vi "LoggingProcess.vi"(0 "Buffers":T3, 5 "FPGA Ref":refnum<k20>, 7 "LoggingIRQ":i32, 11 "error in (no error)":errorcluster, 12 "AnalogLimits":T1) -> ()   [LabVIEW 2015]
uses:
  <vilib>/NI/PowerElectronicsControl/BufferLogging/Buffers.ctl
  <vilib>/NI/PowerElectronicsControl/ScaleAndLimit/Interface/Interface.ctl
  <instrlib>/_niInstr/Instruction Framework/v1/Host/Instruction Target/niInstr Instruction Target v1 Host.lvclass
  <instrlib>/_niInstr/Instruction Framework/v1/Host/Instruction Framework Context/niInstr Instruction Framework Context v1 Host.lvclass
  <vilib>/NI/PowerElectronicsControl/ScaleAndLimit/Interface/Configuration.ctl
  <vilib>/Utility/error.llb/Error Cluster From Error Code.vi
  <vilib>/RVI Host/nirviSupport.llb/nirviErrorClusterFromErrorCode.vi
  <vilib>/rvi/errors/niLvFpgaAdjustHostInterfaceError.vi
  <vilib>/rvi/interface/nirviMethod/nirviMethod.xnode
  <vilib>/rvi/interface/nirviReadWriteControl/nirviReadWriteControl.xnode
  <vilib>/NI/PowerElectronicsControl/BufferLogging/BufferLogging.lvlib
  <vilib>/rvi/interface/nirviMethod/StockFPGA_InlinedMethodWaitForSingleIRQ.vi
  <vilib>/FPGAPlugInAG/Dynamic/niLvFpga_WaitOnIrq_Dynamic.vi
  NiFpgaLv.dll
  <vilib>/rvi/interface/Simulation/niFpgaSimulationCallBeginRW.vi
  <vilib>/FPGAPlugInAG/Dynamic/niLvFpga_AcknowledgeIrq_Dynamic.vi
  <vilib>/NI/PowerElectronicsControl/ScaleAndLimit/Interface/ScaleAndLimitInterface.lvlib
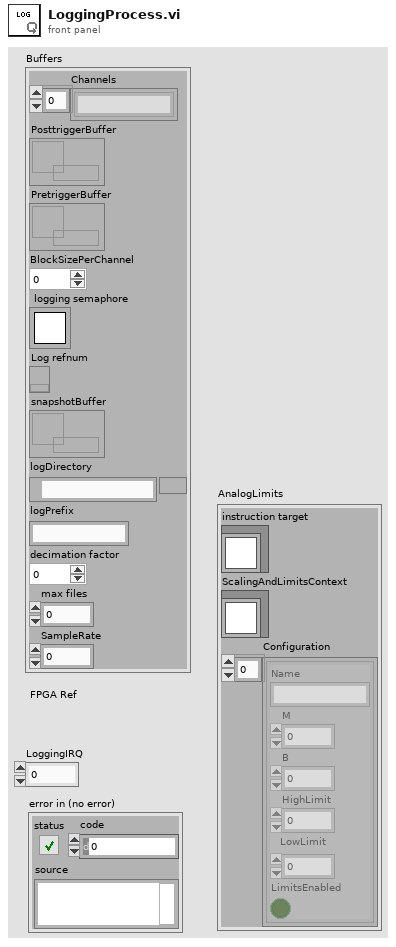
[diagram p1: front panel]
types:
  T1 = typedef "ScaleAndLimitInterface.lvlib/Interface.ctl" = cluster{"instruction target":refnum<class "niInstr Instruction Target v1 Host.lvclass">, "ScalingAndLimitsContext":refnum<class "niInstr Instruction Framework Context v1 Host.lvclass">, "Configuration":T2[]}
  T2 = typedef "ScaleAndLimitInterface.lvlib/Configuration.ctl" = cluster{"Name":string, "M":dbl, "B":i16, "HighLimit":dbl, "LowLimit":dbl, "LimitsEnabled":bool}
  T3 = typedef "BufferLogging.lvlib/Buffers.ctl" = cluster{"Channels":string[], "PosttriggerBuffer":refnum<queue>, "PretriggerBuffer":refnum<queue>, "BlockSizePerChannel":i32, " logging semaphore":T4, "Log refnum":refnum<k34>, "snapshotBuffer":refnum<data-value>, "logDirectory":path, "logPrefix":string, "decimation factor":i32, "max files":i32, "SampleRate":dbl}
  T4 = typedef "Semaphore RefNum" = refnum<k1>
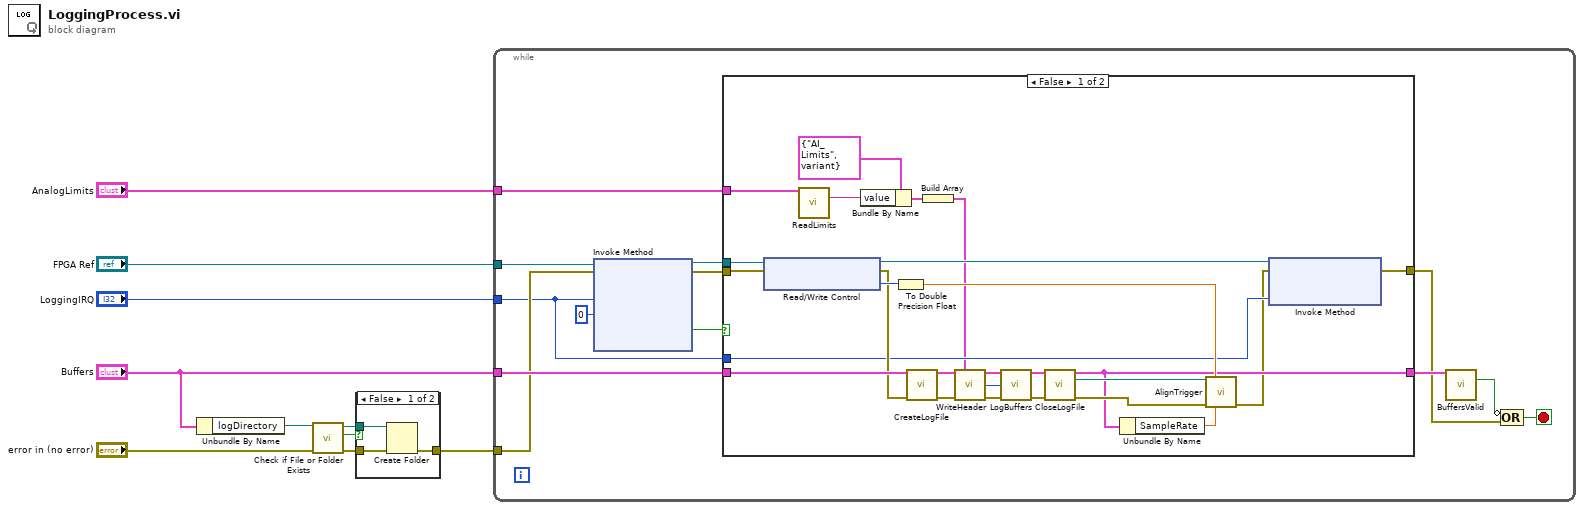
[diagram p0: block diagram]
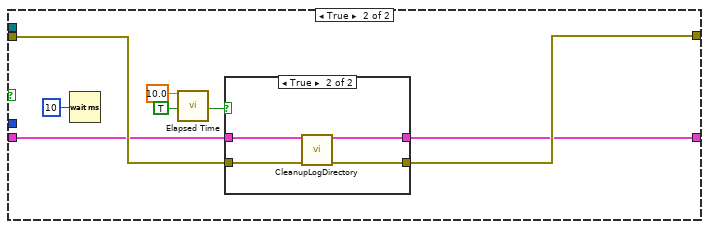
[diagram p3: hidden frame]
diagram:
  n1 = Unbundle By Name("Buffers") -> ("logDirectory"=w9:path)
  n2 = call <vilib>:"Check if File or Folder Exists.vi"("error in (no error)"="error in (no error)", "path"=w9) -> ("error out"=w6:errorcluster, "file or folder exists?"=w8:bool, "dup path"=w5:path)  [unwired: 7 in]
  n3 = case shown="False" w8 {
    tunnel: w6 -> [w12 w14]
    tunnel: w5 -> [w13 _]
    tunnel: [w11 w14] -> w4
    frame False {
      n4 = Create Folder(path (use dialog)=w13, error in=w12) -> (error out=w11:errorcluster)  [unwired: 1 in, 2 out]
    }
    frame True {
    }
  }
  n5 = while {
    tunnel: w4 -> [w20]
    tunnel: "Buffers" -> [w27]
    tunnel: "FPGA Ref" -> [w22]
    tunnel: "LoggingIRQ" -> [w16]
    tunnel: "AnalogLimits" -> [w15]
    stop <- w25 stop-if-true
    n6 = xnode "Invoke Method"("FPGA VI Reference In"=w22, "error in"=w20, "IRQ Number(s)"=w16, "Timeout (ms)"=0) -> ("FPGA VI Reference Out"=w17:refnum<k20>, "error out"=w19:errorcluster, "Timed Out"=w18:bool)  [unwired: 1 out]
    n7 = case shown="False" w18 {
      tunnel: w19 -> [w43 w57]
      tunnel: w27 -> [w53 w55]
      tunnel: [w38 w54] -> w26
      tunnel: [w33 w56] -> w23
      tunnel: w17 -> [w44 _]
      tunnel: w16 -> [w35 _]
      tunnel: w15 -> [w32 _]
      frame False {
        n8 = xnode "Read/Write Control"("FPGA VI Reference In"=w44, "error in"=w43) -> ("FPGA VI Reference Out"=w36:refnum<k20>, "error out"=w40:errorcluster, "TriggerTimestamp"=w42:i32)
        n9 = call <vilib>:"ReadLimits.vi"("Interface in"=w32) -> ("Limits"=w30:string)  [unwired: 12 in, 2 out]
        n10 = Bundle By Name(cluster=cluster{"Property":string, "value":variant} {"Property"="AI_Limits", "value"=variant}, "value"=w30) -> (w29:cluster{"Property":string, "value":variant})
        n11 = To Double Precision Float(number=w42) -> (double precision float=w41:dbl)
        n12 = call <vilib>:"CreateLogFile.vi"("Buffers in"=w53, "error in (no error)"=w40) -> ("Buffers out"=w52:T3, "error out"=w51:errorcluster)  [unwired: 12 in]
        n13 = Build Array(w29) -> (w28:cluster{"Property":string, "value":variant}[])
        n14 = call <vilib>:"WriteHeader.vi"("Buffers in"=w52, "LogMetaData"=w28, "error in (no error)"=w51) -> ("Buffers out"=w50:T3, "numOfChannels"=w48:i32, "error out"=w49:errorcluster)  [unwired: 10 in]
        n15 = call <vilib>:"LogBuffers.vi"("Buffers in"=w50, "numOfChannels"=w48, "error in (no error)"=w49) -> ("Buffers out"=w47:T3, "error out"=w46:errorcluster)  [unwired: 11 in]
        n16 = call <vilib>:"CloseLogFile.vi"("Buffers in"=w47, "error in (no error)"=w46) -> ("Buffers out"=w38:T3, "log path out"=w45:path, "error out"=w39:errorcluster)  [unwired: 11 in]
        n17 = Unbundle By Name(w38) -> ("SampleRate"=w37:dbl)
        n18 = call <vilib>:"AlignTrigger.vi"("log path in"=w45, "triggerTimestamp"=w41, "error in (no error)"=w39, "AcqRate"=w37) -> ("error out"=w34:errorcluster)  [unwired: 10 in, 1 out]
        n19 = xnode "Invoke Method"("FPGA VI Reference In"=w36, "error in"=w34, "IRQ Number(s)"=w35) -> ("error out"=w33:errorcluster)  [unwired: 1 out]
      }
      frame True {
        n20 = Wait (ms)(milliseconds to wait=u32 10) -> ()  [unwired: 1 out]
        n21 = call "Elapsed Time"("Time Target (s)"=10.0, "Auto Reset"=TRUE) -> ("Time has Elapsed"=w58:bool)  [unwired: 10 in, 7 out]
        n22 = case shown="True" w58 {
          tunnel: w57 -> [w63 w67]
          tunnel: [w63 w66] -> w56
          tunnel: w55 -> [w62 w65]
          tunnel: [w62 w64] -> w54
          frame False {
          }
          frame True {
            n23 = call <vilib>:"CleanupLogDirectory.vi"("BuffersIn"=w65, "error in"=w67) -> ("BuffersOut"=w64:T3, "error out"=w66:errorcluster)  [unwired: 12 in]
          }
        }
      }
    }
    n24 = call <vilib>:"BuffersValid.vi"("Buffers in"=w26) -> ("valid"=w24:bool)  [unwired: 13 in, 1 out]
    n25 = Compound Arithmetic op=OR(invert w24, w23) -> (w25:bool)
  }
